vi "KE622x -- Get Arm Source.vi"(0 "Resource In":refnum<visa-resource-name>, 1 "Check For SCPI Errors? (T)":bool=TRUE, 11 "error in (no error)":errorcluster) -> (4 "Resource Out (dupl)":refnum<visa-resource-name>, 8 "Arm Source":T1, 15 "error out":errorcluster)   [LabVIEW 2018, in "Keithley 622x.lvlib"]
uses:
  Keithley 622x.lvlib
  Typedefs/KE622x -- Arm Source.ctl
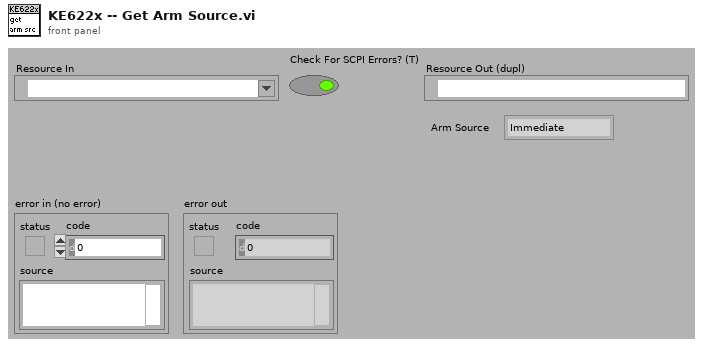
[diagram p1: front panel]
types:
  T1 = typedef "Keithley 622x.lvlib/KE622x -- Arm Source.ctl" = enum16{"Immediate", "Bus (*TRG)", "Timer", "Manual", "Trigger Link", "SOT Falling Edge", "SOT Rising Edge", "SOT Either Edge"}
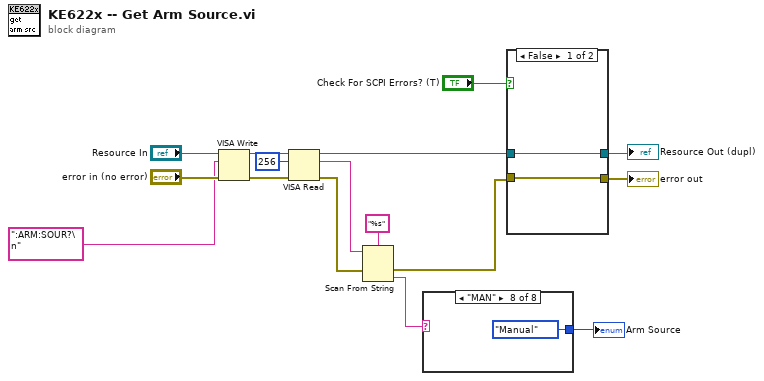
[diagram p0: block diagram]
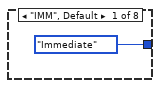
[diagram p2: hidden frame]
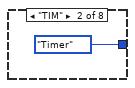
[diagram p3: hidden frame]
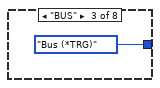
[diagram p4: hidden frame]
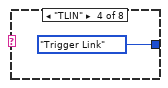
[diagram p5: hidden frame]
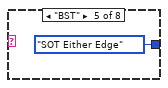
[diagram p6: hidden frame]
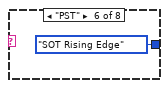
[diagram p7: hidden frame]
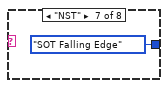
[diagram p8: hidden frame]
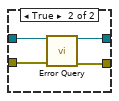
[diagram p9: hidden frame]
diagram:
  n1 = VISA Write(VISA resource name="Resource In", write buffer=":ARM:SOUR?\n" ("format string"), error in (no error)="error in (no error)") -> (VISA resource name out=w10:refnum<visa-resource-name>, error out=w9:errorcluster)  [unwired: 1 out]
  n2 = VISA Read(VISA resource name=w10, byte count=u32 256, error in (no error)=w9) -> (VISA resource name out=w3:refnum<visa-resource-name>, read buffer=w5:string, error out=w7:errorcluster)  [unwired: 1 out]
  n3 = Scan From String(format string="%s", input string=w5, error in=w7) -> (error out=w4:errorcluster, output 1=w2:string)  [unwired: 2 in, 2 out]
  n4 = case shown="\"MAN\"" w2 {
    tunnel: [KE622x_--_Arm_Source."Immediate" ("Arm-In Source") KE622x_--_Arm_Source."Timer" ("Arm-In Source") KE622x_--_Arm_Source."Bus (*TRG)" ("Arm-In Source") KE622x_--_Arm_Source."Trigger Link" ("Arm-In Source") KE622x_--_Arm_Source."SOT Either Edge" ("Arm-In Source") KE622x_--_Arm_Source."SOT Rising Edge" ("Arm-In Source") KE622x_--_Arm_Source."SOT Falling Edge" ("Arm-In Source") KE622x_--_Arm_Source."Manual" ("Arm-In Source")] -> w1
    frame "IMM", Default {
    }
    frame "TIM" {
    }
    frame "BUS" {
    }
    frame "TLIN" {
    }
    frame "BST" {
    }
    frame "PST" {
    }
    frame "NST" {
    }
    frame "MAN" {
    }
  }
  "Arm Source" <- w1
  n5 = case shown="False" "Check For SCPI Errors? (T)" {
    tunnel: w3 -> [w26 w30]
    tunnel: w4 -> [w25 w29]
    tunnel: [w25 w28] -> w12
    tunnel: [w26 w27] -> w13
    frame False {
    }
    frame True {
      n6 = call "Error Query.vi"("VISA Resource In"=w30, "error in (no error)"=w29) -> ("VISA Resource Out (dupl)"=w27:refnum<visa-resource-name>, "error out"=w28:errorcluster)  [unwired: 10 in, 2 out]
    }
  }
  "Resource Out (dupl)" <- w13
  "error out" <- w12
